vi "MARS_Set_Auto_properties_wrapper.vi"(6 "Total Time":dbl, 8 "error in (no error)":errorcluster, 9 "Channel name":string[](array[string]), 10 "group name in":string, 11 "Refnum in":refnum<k34>) -> (0 "error out":errorcluster, 3 "Refnum out":refnum<k34>)   [LabVIEW 2015]
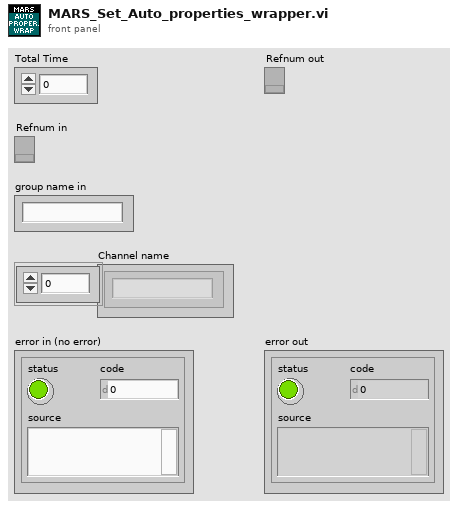
[diagram p1: front panel]
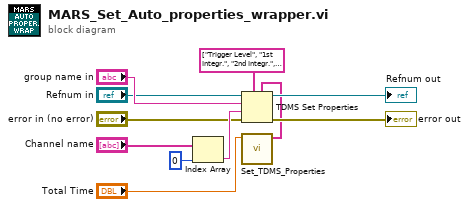
[diagram p0: block diagram]
diagram:
  n1 = Index Array(array="Channel name", index=0) -> (element=w11:string)
  n2 = call "Set_TDMS_Properties.vi"("Total time"="Total Time") -> ("TDMS Properties"=w4:string[])  [unwired: 10 in]
  n3 = TDMS Set Properties(5:w4, 7:string[] ["Trigger Level", "1st Integr.", "2nd Integr.", "Duration"] ("property names"), 8:"error in (no error)", 9:w11, 10:"group name in", 11:"Refnum in") -> (0:→"error out":errorcluster, 3:→"Refnum out":refnum<k34>)  [unwired: 2 out]
